vi "Null To String.vi"(7 "enable LabVIEW extensions? (T)":bool=TRUE, 8 "error in (no error)":errorcluster, 11 "JSON Datatype in":refnum<class "JSON Helper.lvclass">) -> (0 "error out":errorcluster, 3 "String":string)   [LabVIEW 2016, in "JSON Helper.lvclass"]
doc: "Flattens the given JSON data to a string."
uses:
  JSON Helper/JSON Helper.lvclass
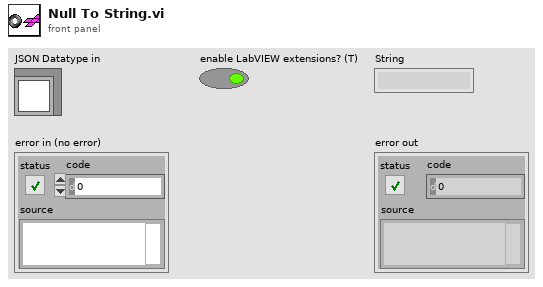
[diagram p1: front panel]
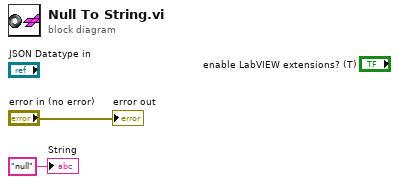
[diagram p0: block diagram]
diagram:
  "String" <- "null" ("String")
  "error out" <- "error in (no error)"
